vi "Compute Start Postion in one line.vi"(7 "error in (no error)":errorcluster, 8 "original position":cluster{"row":i8, "column":i8}, 9 "string length in":i32, 10 "cluster of private data in":T1={"FPGA VI Reference"=refnum, "device index"=0, "screen size"=enum."8x1", "font size"=enum."5x8", "auto wrap"=FALSE, "alignment"=enum."None", "number of line"=enum."2 lines", "shift 0"=0, "entry mode 0"=enum."increment & no shift", "shift 1"=0, "entry mode 1"=enum."increment & no shift"}) -> (0 "error out":errorcluster, 1 "output position":cluster{"row":i8, "column":i8}, 2 "string length out":i32, 3 "cluster of private data out":T1={"FPGA VI Reference"=refnum, "device index"=0, "screen size"=enum."8x1", "font size"=enum."5x8", "auto wrap"=FALSE, "alignment"=enum."None", "number of line"=enum."2 lines", "shift 0"=0, "entry mode 0"=enum."increment & no shift", "shift 1"=0, "entry mode 1"=enum."increment & no shift"})   [LabVIEW 2017, in "HD44780.lvclass"]
uses:
  HD44780.lvclass
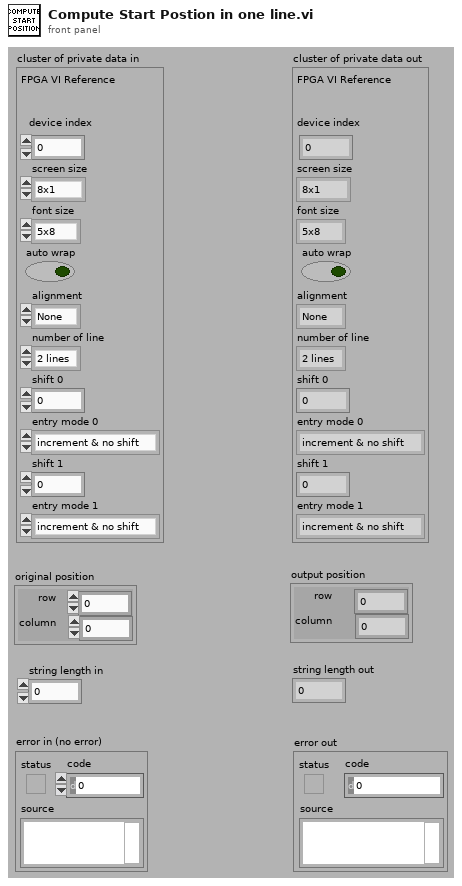
[diagram p1: front panel]
types:
  T1 = cluster{"FPGA VI Reference":refnum<k20>, "device index":i8, "screen size":enum8{"8x1", "8x2", "12x4", "16x1", "16x2", "16x4", "20x1", "20x2", "20x4", "24x1", "24x2", "40x2", "40x4"}, "font size":enum8{"5x8", "5x10"}, "auto wrap":bool, "alignment":enum16{"None", "Left", "Center", "Right"}, "number of line":enum8{"1 line", "2 lines"}, "shift 0":i8, "entry mode 0":enum8{"increment & no shift", "increment & shift", "decrement & no shift", "decrement & shift"}, "shift 1":i8, "entry mode 1":enum8{"increment & no shift", "increment & shift", "decrement & no shift", "decrement & shift"}}
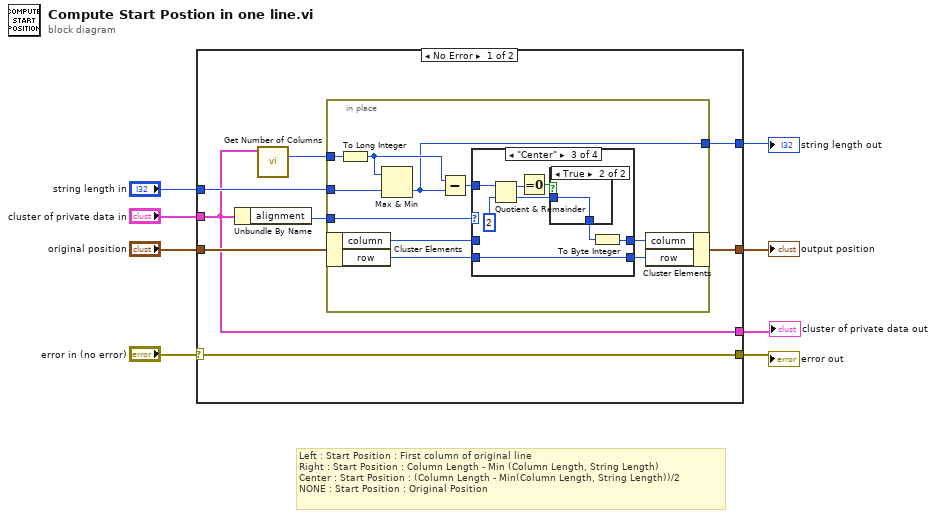
[diagram p0: block diagram]
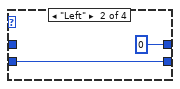
[diagram p3: hidden frame]
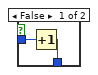
[diagram p4: hidden frame]
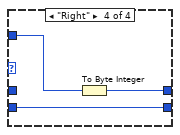
[diagram p5: hidden frame]
diagram:
  # "Left : Start Position : First column of original line\nRight : Start Position : Column Length - Min (Column Length, String Length)\nCenter : Start Position : (Column Length - Min(Column Length, String Length))/2\nNONE : Start Position : Original Position"
  n1 = case shown="No Error" "error in (no error)" {
    selector: "error in (no error)" -> [w9 w46]
    tunnel: "string length in" -> [w16 w48]
    tunnel: "original position" -> [w15 w47]
    tunnel: [w14 w47] -> w6
    tunnel: [w13 w48] -> w5
    tunnel: "cluster of private data in" -> [w10 w45]
    tunnel: [w10 w45] -> w2
    tunnel: [w9 w46] -> w1
    frame No Error {
      n2 = Unbundle By Name(w10) -> ("alignment"=w11:enum16{"None", "Left", "Center", "Right"})
      n3 = call "Get Number of Columns.vi"("cluster of private data in"=w10) -> ("column number"=w12:u8)  [unwired: 10 in]
      n4 = in-place {
        in-place-border: w16 -> [w21]
        in-place-border: w12 -> [w22]
        in-place-border: [w19] -> w13
        in-place-border: w11 -> [w17]
        n5 = in-place-cluster #1(w15) -> ("column"=w24:i8, "row"=w26:i8)
        n6 = To Long Integer(number=w22) -> (32bit integer=w20:i32)
        n7 = Max & Min(x=w20, y=w21) -> (min(x,y)=w19:i32)  [unwired: 1 out]
        n8 = Subtract(x=w20, y=w19) -> (x-y=w18:i32)
        n9 = case shown="\"Center\"" w17 {
          tunnel: w24 -> [w27 _ _ _]
          tunnel: [w28 w30 w38 w44] -> w25
          tunnel: w26 -> [w28 w30 w38 w44]
          tunnel: [w27 i8 0 ("column") w31 w43] -> w23
          tunnel: w18 -> [_ _ w37 w42]
          frame "None", Default {
          }
          frame "Left" {
          }
          frame "Center" {
            n10 = Quotient & Remainder(x=w37, y=2) -> (x-y*floor(x/y)=w35:i32, floor(x/y)=w33:i32)
            n11 = Equal To 0?(x=w35) -> (x = 0?=w34:bool)
            n12 = case shown="True" w34 {
              tunnel: w33 -> [w40 w41]
              tunnel: [w39 w41] -> w32
              frame False {
                n13 = Increment(x=w40) -> (x+1=w39:i32)
              }
              frame True {
              }
            }
            n14 = To Byte Integer(number=w32) -> (8bit integer=w31:i8)
          }
          frame "Right" {
            n15 = To Byte Integer(number=w42) -> (8bit integer=w43:i8)
          }
        }
        n16 = in-place-cluster #1("column"=w23, "row"=w25) -> (w14:cluster{"row":i8, "column":i8})
      }
    }
    frame Error {
    }
  }
  "output position" <- w6
  "error out" <- w1
  "string length out" <- w5
  "cluster of private data out" <- w2
